vi "zadanie6_1.vi"() -> ()   [LabVIEW 2012]
panel:
  in  "Oblicz":bool
  in  "Drugi wyraz ciągu arytmetycznego:":i32
  in  "Pierwszy wyraz ciągu arytmetycznego:":i32
  out "Użytkownik:":string
  out "Wyrazy ciągu arytmetycznego":i32[][](array[numeric])
  # "Program oblicza kolejne wyrazy ciągu arytmetycznego na podstawie podanego pierwszego i drugiego wyrazu tego ciągu"
  # "numer wyrazu:"
  # "wartość:"
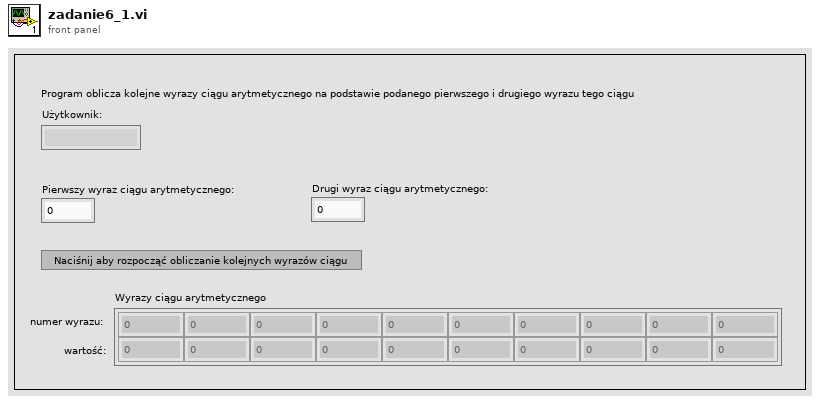
[diagram p1: front panel]
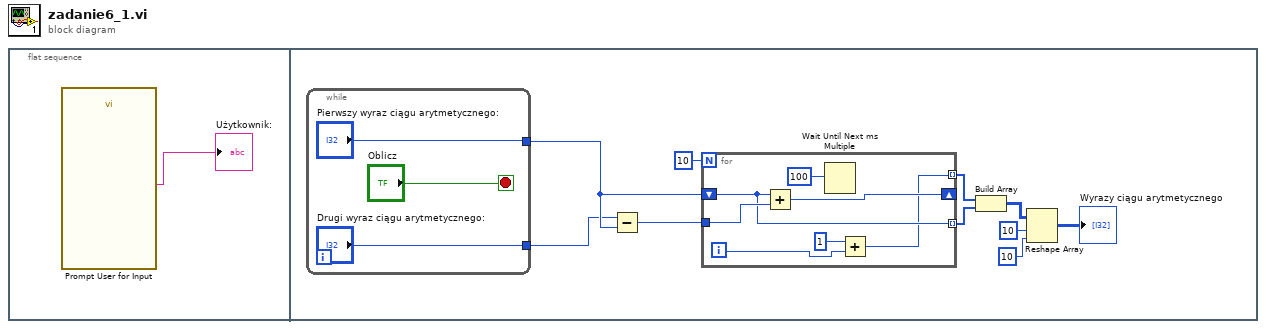
[diagram p0: block diagram]
diagram:
  n1 = flat-sequence {
    frame #0 {
      n2 = call "Prompt User for Input"() -> ("Login"=→"Użytkownik:":string)  [unwired: 16 in, 3 out]
    }
    frame #1 {
      n3 = while {
        tunnel: ["Pierwszy wyraz ciągu arytmetycznego:"] -> w4
        tunnel: ["Drugi wyraz ciągu arytmetycznego:"] -> w2
        stop <- "Oblicz" stop-if-true
      }
      n4 = Subtract(x=w2, y=w4) -> (x-y=w5:i32)
      n5 = for {
        N: 10 -> [_]
        tunnel: w5 -> [w21]
        shift-right: [w20] -> _
        shift-left: w4 -> [w19]
        tunnel: [w19] -> w8 mode=indexing
        tunnel: [w18] -> w11 mode=indexing
        i -> [w16]
        n6 = Add(x=w19, y=w21) -> (x+y=w20:i32)
        n7 = Wait Until Next ms Multiple(millisecond multiple=100) -> ()  [unwired: 1 out]
        n8 = Add(x=1, y=w16) -> (x+y=w18:i32)
      }
      n9 = Build Array(w11, w8) -> (w7:i32[][])
      n10 = Reshape Array(w7, 10 ("dimension size"), 10 ("dimension size")) -> (→"Wyrazy ciągu arytmetycznego":i32[][])
    }
  }
